vi "Read From Disk.vi"(8 "error in (no error)":errorcluster, 11 "csv-formatter in":refnum<class "csv-formatter.lvclass">) -> (0 "error out":errorcluster, 2 "Result Out":string[][](array[string]), 3 "csv-formatter out":refnum<class "csv-formatter.lvclass">)   [LabVIEW 2015, in "csv-formatter.lvclass"]
uses:
  csv-formatter.lvclass
  csv-formatter.lvclass/csv-formatter.ctl
  <vilib>/Utility/file.llb/Read Delimited Spreadsheet (string).vi
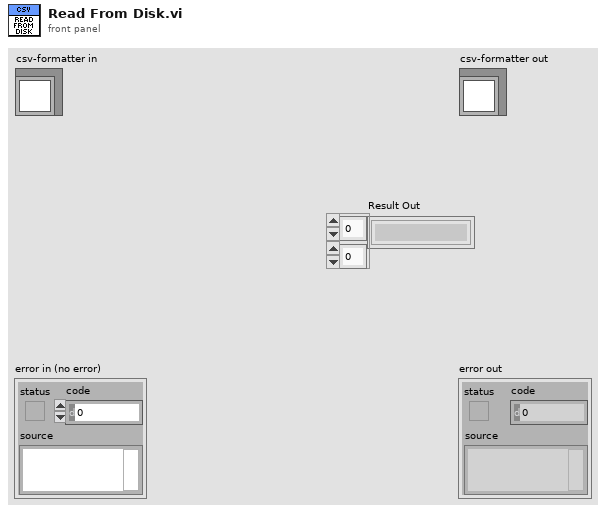
[diagram p1: front panel]
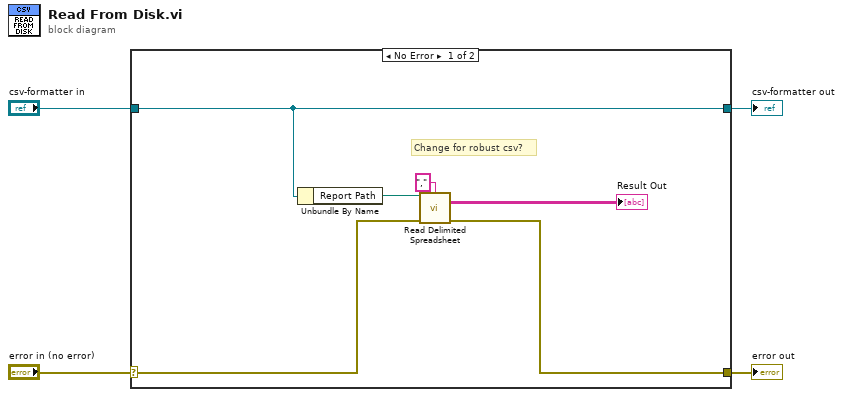
[diagram p0: block diagram]
diagram:
  n1 = case shown="No Error" "error in (no error)" {
    selector: "error in (no error)" -> [w6 w12]
    tunnel: [w5 w12] -> w3
    tunnel: [w10 w11] -> w1
    tunnel: "csv-formatter in" -> [w10 w11]
    frame No Error {
      # "Change for robust csv?"
      n2 = Unbundle By Name(w10) -> ("Report Path"=w9:path)
      n3 = call-poly <vilib>:"Read Delimited Spreadsheet.vi"("file path (dialog if empty)"=w9, "error in (no error)"=w6, "delimiter (\\t)"="," ("delimiter (\\t)")) -> ("all rows"=→"Result Out":string[][], "error out"=w5:errorcluster)  [unwired: 7 in, 4 out]
    }
    frame Error {
    }
  }
  "error out" <- w3
  "csv-formatter out" <- w1
